vi "G#Object_GenericCreate.vi"(0 "class path":path, 2 "control names":string[](array[string]), 3 "control values":variant[](array[variant]), 4 "timeout in ms (-1)":i32=-1, 5 "error in (no error)":errorcluster, 6 "keep constructor VI ref open? (T)":bool=TRUE, 7 "respond to create event? (T)":bool=TRUE) -> (12 "constructor VI ref":refnum<vi>, 14 "reference out":refnum<class "G#Object.lvclass">, 19 "error out":errorcluster)   [LabVIEW 2020, in "G#Object.lvclass"]
doc: "Creates an instance of the class specified by the path. The path could either be directly to the constructor method, the .lvclass file or to the class folder. It is also possible to set the constructor input parameters by the \"Control Names\" and \"Control Values\" inputs.\n\nSince this function runs the constructor with VI server, making the constructor \"running top-level\", it is necessary to use the external create event in order to let this VI create the needed object and become the owner of the queues and data value reference. However, if the constructor also contains user defined queues, notifiers etc., these will be garbage collected by LabVIEW when the constructor is finished executing. To avoid this, use the Default Constructor instead.\n\nBe careful when using this VI when building executables, since paths must be correct and make sure that all needed VIs are included in the build.\n\nNote: Will not work on RT systems."
uses:
  G#Object.lvclass
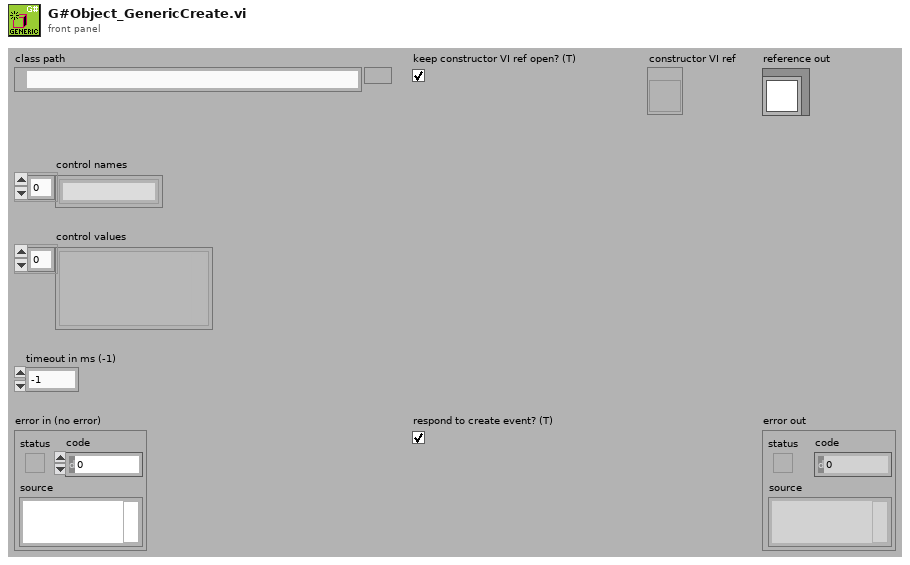
[diagram p1: front panel]
types:
  T1 = typedef "G#Object.lvclass/G#Object_EventType.ctl" = enum16{"Created new", "Looked up existing", "Deleted", "Forced delete", "Not deleted", "Garbage collected", "Cleared", "User", "Error", "External create object", "External create class attributes", "Created class attributes", "Run constructor", "Run constructor done", "Run open method", "Run open method done"}
  T2 = typedef "G#Object.lvclass/G#Object_ObjectInfoType.ctl" = cluster{"ObjectName":string, "ObjectID":u32, "Users":i32, "Counter":bool, "AttributeRefs":u32[], "FullClassName":string, "ClassName":string, "CreateMethod":T3, "GenericDestructorExists":bool, "Owner":string}
  T3 = typedef "G#Object.lvclass/G#Object_CreateMethod.ctl" = enum16{"Create", "Create or look up existing", "Look up existing"}
  T4 = enum32{"Bad", "Idle", "Run top level", "Running"}
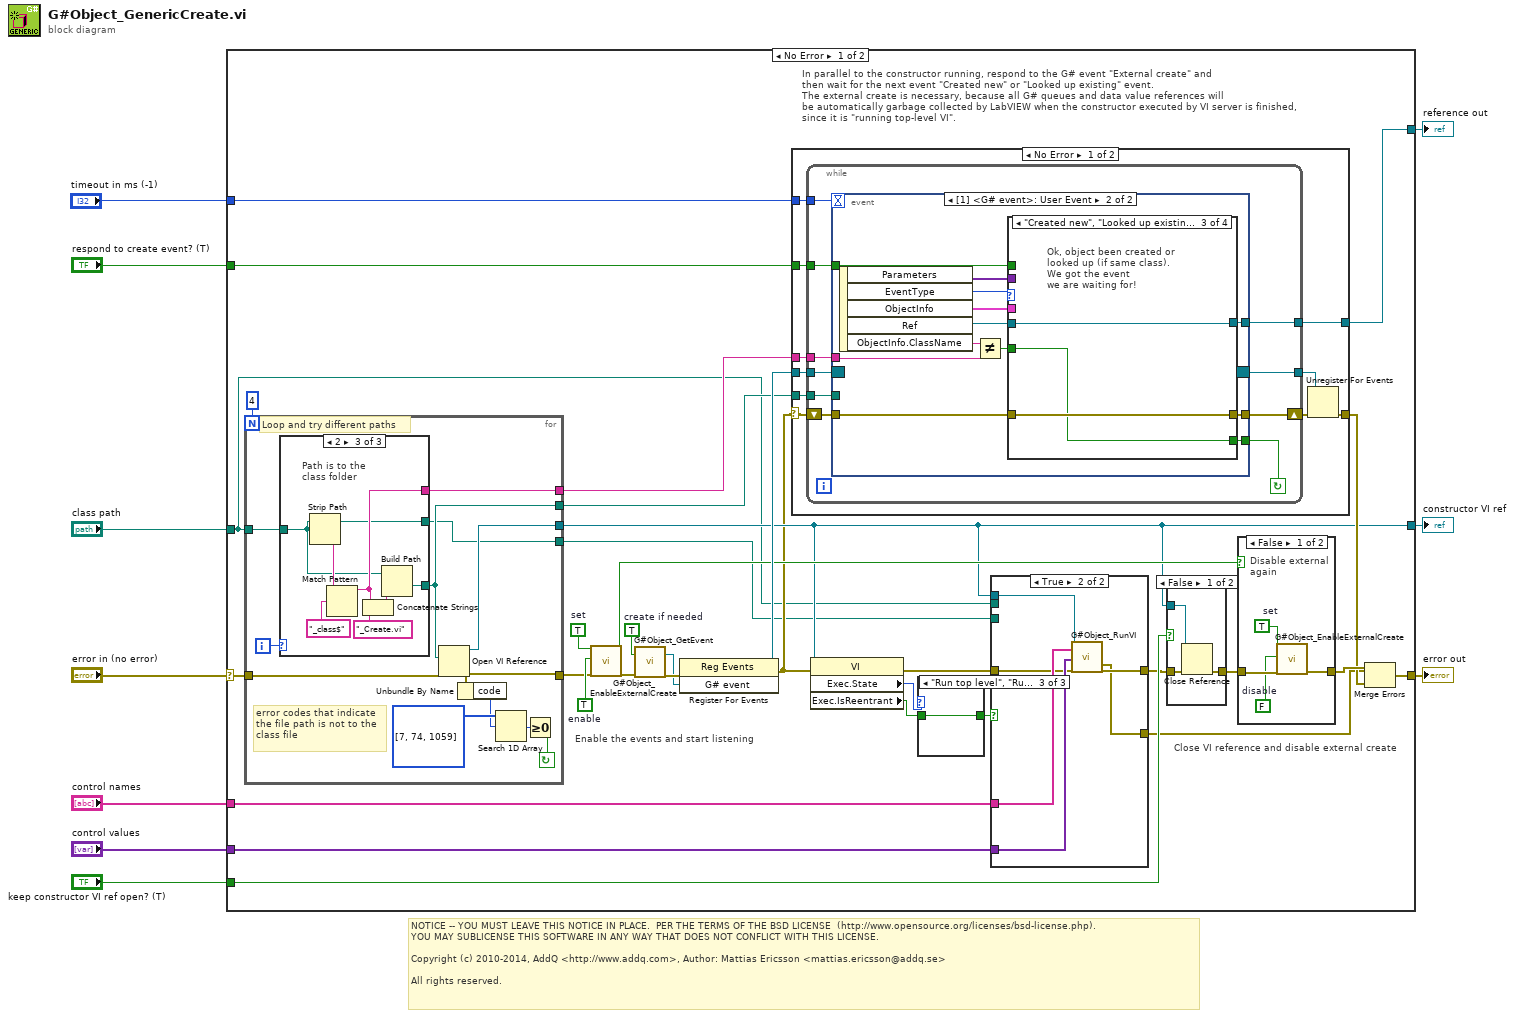
[diagram p0: block diagram]
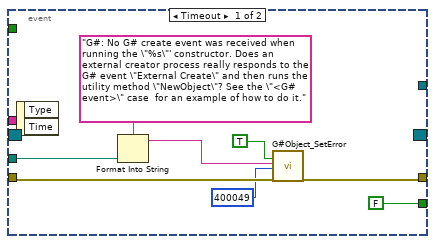
[diagram p2: hidden frame]
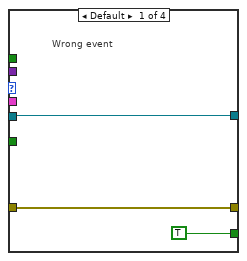
[diagram p3: hidden frame]
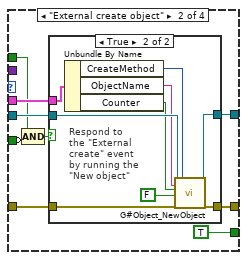
[diagram p4: hidden frame]
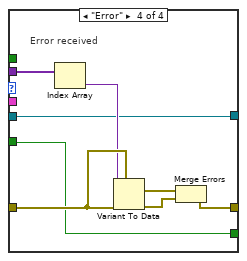
[diagram p6: hidden frame]
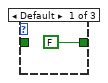
[diagram p8: hidden frame]
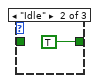
[diagram p9: hidden frame]
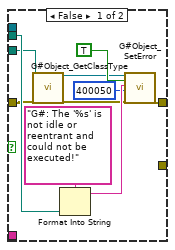
[diagram p10: hidden frame]
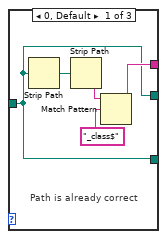
[diagram p13: hidden frame]
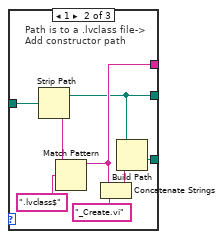
[diagram p14: hidden frame]
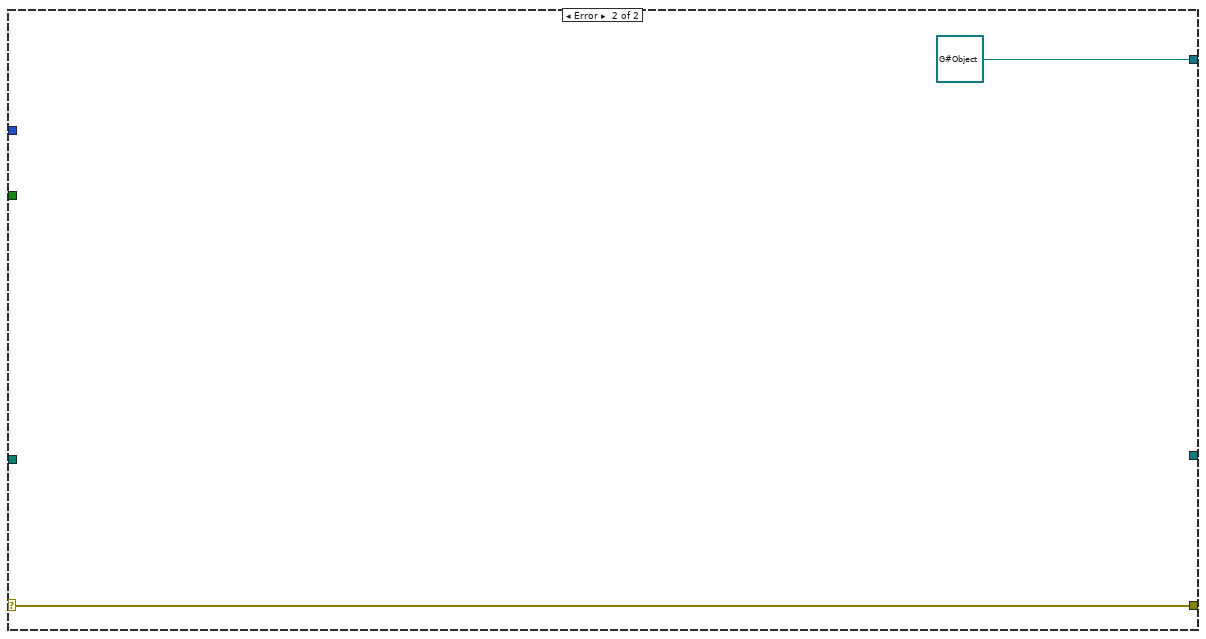
[diagram p15: hidden frame]
diagram:
  # "NOTICE -- YOU MUST LEAVE THIS NOTICE IN PLACE.  PER THE TERMS OF THE BSD LICENSE  (http://www.opensource.org/licenses/bsd-license.php).\nYOU MAY SUBLICENSE THIS SOFTWARE IN ANY WAY THAT DOES NOT CONFLICT WITH THIS LICENSE.\n\nCopyright (c) 2010-2014, AddQ <http://www.addq.com>, Author: Mattias Ericsson <mattias.ericsson@addq.se>\n\nAll rights reserved."
  n1 = case shown="No Error" "error in (no error)" {
    selector: "error in (no error)" -> [w25 w180]
    tunnel: [w36 w180] -> w9
    tunnel: [w37 refnum<class "G#Object.lvclass"> refnum ("reference in (for type)")] -> w8
    tunnel: "control names" -> [w43 _]
    tunnel: "control values" -> [w42 _]
    tunnel: "class path" -> [w12 _]
    tunnel: "keep constructor VI ref open? (T)" -> [w35 _]
    tunnel: [w19 _] -> w3
    tunnel: "respond to create event? (T)" -> [w34 _]
    tunnel: "timeout in ms (-1)" -> [w14 _]
    frame No Error {
      w31 = TRUE  # enable
      w32 = TRUE  # set
      w28 = TRUE  # create if needed
      # "Enable the events and start listening"
      # "Close VI reference and disable external create"
      # "In parallel to the constructor running, respond to the G# event \"External create\" and\nthen wait for the next event \"Created new\" or \"Looked up existing\" event.\nThe external create is necessary, because all G# queues and data value references will\nbe automatically garbage collected by LabVIEW when the constructor executed by VI server is finished,\nsince it is \"running top-level VI\"."
      n2 = for {
        N: 4 -> [_]
        tunnel: w12 -> [w157]
        tunnel: [w156] -> w19
        tunnel: [w155] -> w15
        tunnel: [w154] -> w27
        tunnel: [w147] -> w26
        tunnel: w25 -> [w153]
        tunnel: [w152] -> w11
        i -> [w158]
        stop <- w148 continue-if-true
        # "error codes that indicate\nthe file path is not to the\nclass file"
        # "Loop and try different paths"
        n3 = case shown="2" w158 {
          tunnel: w157 -> [w159 w171 w172]
          tunnel: [w159 w166 w174] -> w155
          tunnel: [w160 w165 w173] -> w154
          tunnel: [w159 w164 w172] -> w152
          frame 0, Default {
            # "Path is already correct"
            n4 = Strip Path(path=w159) -> (stripped path=w161:path)  [unwired: 1 out]
            n5 = Strip Path(path=w161) -> (name=w163:string)  [unwired: 1 out]
            n6 = Match Pattern(string=w163, regular expression="_class$") -> (before substring=w160:string)  [unwired: 1 in, 3 out]
          }
          frame 1 {
            # "Path is to a .lvclass file->\nAdd constructor path"
            n7 = Strip Path(path=w171) -> (stripped path=w164:path, name=w170:string)
            n8 = Match Pattern(string=w170, regular expression=".lvclass$") -> (before substring=w165:string)  [unwired: 1 in, 3 out]
            n9 = Concatenate Strings(w165, "_Create.vi" ("string")) -> (w167:string)
            n10 = Build Path(base path=w164, name or relative path=w167) -> (appended path=w166:path)
          }
          frame 2 {
            # "Path is to the \nclass folder"
            n11 = Strip Path(path=w172) -> (name=w178:string)  [unwired: 1 out]
            n12 = Match Pattern(string=w178, regular expression="_class$") -> (before substring=w173:string)  [unwired: 1 in, 3 out]
            n13 = Concatenate Strings(w173, "_Create.vi" ("string")) -> (w175:string)
            n14 = Build Path(base path=w172, name or relative path=w175) -> (appended path=w174:path)
          }
        }
        n15 = Open VI Reference(vi path=w155, error in (no error)=w153) -> (vi reference=w156:refnum<vi>, error out=w147:errorcluster)  [unwired: 4 in]
        n16 = Unbundle By Name(w147) -> ("code"=w149:i32)
        n17 = Search 1D Array(1D array=i32[] [7, 74, 1059], element=w149) -> (index of element=w151:i32)  [unwired: 1 in]
        n18 = Greater Or Equal To 0?(x=w151) -> (x >= 0?=w148:bool)
      }
      n19 = call "G#Object_EnableExternalCreate.vi"("set (F)"=w32, "external create enable (F)"=w31, "error in (no error)"=w26) -> ("already enabled"=w29:bool, "error out"=w33:errorcluster)  [unwired: 14 in, 1 out]
      n20 = call "G#Object_GetEvent.vi"("create if needed (T)"=w28, "error in (no error)"=w33) -> ("G# event"=w39:refnum<user-event>, "error out"=w40:errorcluster)  [unwired: 13 in, 3 out]
      n21 = register-events(error in=w40, w39) -> (reference out=w38:refnum<event-registration>, error out=w13:errorcluster)  [unwired: 1 in]
      n22 = case shown="No Error" w13 {
        selector: w13 -> [w44 w118]
        tunnel: w38 -> [w53 _]
        tunnel: [w52 _] -> w37
        tunnel: w34 -> [w49 _]
        tunnel: w27 -> [w48 _]
        tunnel: [w47 w118] -> w23
        tunnel: w15 -> [w46 _]
        tunnel: w14 -> [w45 _]
        frame No Error {
          n23 = while {
            tunnel: w53 -> [w63]
            shift-right: [w61] -> w51
            shift-left: w44 -> [w62]
            tunnel: [w59] -> w52
            tunnel: [w58] -> w50
            tunnel: w49 -> [w57]
            tunnel: w46 -> [w56]
            tunnel: w48 -> [w55]
            tunnel: w45 -> [w54]
            stop <- w60 continue-if-true
            n24 = event shown="[1] <G# event>: User Event" {
              selector: w63 -> [_ _]
              dyn-events: [_ _] -> w58
              timeout: w54 -> [_ _]
              tunnel: w62 -> [w69 w82]
              tunnel: [w70 w79] -> w61
              tunnel: [FALSE w78] -> w60
              tunnel: [_ w77] -> w59
              tunnel: w57 -> [_ w76]
              tunnel: w56 -> [w65 _]
              tunnel: w55 -> [_ w74]
              event Timeout {
                n25 = event-data() -> ()  [unwired: 1 in, 2 out]
                n26 = Format Into String(format string="G#: No G# create event was received when running the \"%s\"' constructor. Does an external creator process really responds to the G# event \"External Create\" and then runs the utility method \"NewObject\"? See the \"<G# event>\" case  for an example of how to do it." ("source"), w65) -> (resulting string=w66:string)  [unwired: 2 in, 1 out]
                n27 = call "G#Object_SetError.vi"("error (F)"=TRUE ("error"), "source"=w66, "code"=400049, "error in (no error)"=w69) -> ("error out"=w70:errorcluster)  [unwired: 15 in]
              }
              event User Event {
                n28 = event-data() -> ("Parameters"=w72:variant[], "EventType"=w83:T1, "ObjectInfo"=w81:T2, "Ref"=w80:refnum<class "G#Object.lvclass">, "ObjectInfo.ClassName"=w75:string)  [unwired: 1 in]
                n29 = Not Equal?(x=w75, y=w74) -> (x != y?=w73:bool)
                n30 = case shown="\"Created new\", \"Looked up existing\"" w83 {
                  tunnel: w82 -> [w85 w95 w109 w117]
                  tunnel: w81 -> [_ w92 _ _]
                  tunnel: w80 -> [w86 w91 w108 w111]
                  tunnel: [w85 w94 w109 w114] -> w79
                  tunnel: [TRUE TRUE w107 w110] -> w78
                  tunnel: [w86 w90 w108 w111] -> w77
                  tunnel: w76 -> [_ w88 _ _]
                  tunnel: w73 -> [_ w89 w107 w110]
                  tunnel: w72 -> [_ _ _ w116]
                  frame Default {
                    # "Wrong event"
                  }
                  frame "External create object" {
                    n31 = Compound Arithmetic op=AND(w88, invert w89) -> (w87:bool)
                    n32 = case shown="True" w87 {
                      tunnel: w95 -> [w96 w106]
                      tunnel: [w96 w105] -> w94
                      tunnel: w92 -> [_ w104]
                      tunnel: w91 -> [w97 w103]
                      tunnel: [w97 w102] -> w90
                      frame False {
                        # "Don't respond to external\ncreate event"
                      }
                      frame True {
                        # "Respond to\nthe \"External\ncreate\" event\nby running the\n\"New object\""
                        n33 = Unbundle By Name(w104) -> ("CreateMethod"=w101:T3, "ObjectName"=w100:string, "Counter"=w99:bool)
                        n34 = call "G#Object_NewObject.vi"("reference in"=w103, "object name (\"\")"=w100, "user counter (T)"=w99, "no registration (F)"=FALSE ("no registration"), "error in (no error)"=w106, "create method"=w101) -> ("reference out"=w102:refnum<class "G#Object.lvclass">, "error out"=w105:errorcluster)  [unwired: 11 in, 1 out]
                      }
                    }
                  }
                  frame "Created new", "Looked up existing" {
                    # "Ok, object been created or \nlooked up (if same class).\nWe got the event\nwe are waiting for!"
                  }
                  frame "Error" {
                    # "Error received"
                    n35 = Index Array(array=w116) -> (element=w115:variant)  [unwired: 1 in]
                    n36 = Variant To Data(error in=w117, type=w117, Variant=w115) -> (data=w112:errorcluster, error out=w113:errorcluster)
                    n37 = Merge Errors(w112, w113) -> (w114:errorcluster)
                  }
                }
              }
            }
          }
          n38 = Unregister For Events(event registration refnum=w50, error in=w51) -> (error out=w47:errorcluster)
        }
        frame Error {
        }
      }
      n39 = property class="VI"(reference=w19, error in=w13) -> (error out=w22:errorcluster, "Exec.State"=w18:T4, "Exec.IsReentrant"=w16:bool)  [unwired: 1 out]
      n40 = case shown="\"Run top level\", \"Running\"" w18 {
        tunnel: [FALSE TRUE w121] -> w17
        tunnel: w16 -> [_ _ w121]
        frame Default {
        }
        frame "Idle" {
        }
        frame "Run top level", "Running" {
        }
      }
      n41 = case shown="True" w17 {
        tunnel: w43 -> [_ w137]
        tunnel: w42 -> [_ w136]
        tunnel: w22 -> [w125 w135]
        tunnel: [w131 w134] -> w21
        tunnel: [_ w133] -> w20
        tunnel: w19 -> [_ w132]
        tunnel: w12 -> [w128 _]
        tunnel: w11 -> [w123 _]
        frame False {
          n42 = call "G#Object_GetClassType.vi"("class path"=w123, "error in (no error)"=w125) -> ("reference out"=w122:refnum<class "G#Object.lvclass">, "error out"=w124:errorcluster)  [unwired: 16 in]
          n43 = Format Into String(format string="G#: The '%s' is not idle or reentrant and could not be executed!", w128) -> (resulting string=w127:string)  [unwired: 2 in, 1 out]
          n44 = call "G#Object_SetError.vi"("reference in"=w122, "error (F)"=TRUE ("error"), "source"=w127, "code"=400050, "error in (no error)"=w124) -> ("error out"=w131:errorcluster)  [unwired: 14 in]
        }
        frame True {
          n45 = call "G#Object_RunVI.vi"("vi reference"=w132, "control names"=w137, "control values"=w136, "error in (no error)"=w135) -> ("error out from VI"=w133:errorcluster, "error out"=w134:errorcluster)  [unwired: 14 in]
        }
      }
      n46 = case shown="False" w35 {
        tunnel: w21 -> [w145 w146]
        tunnel: w19 -> [w143 _]
        tunnel: [w144 w146] -> w30
        frame False {
          n47 = Close Reference(reference=w143, error in (no error)=w145) -> (error out=w144:errorcluster)
        }
        frame True {
        }
      }
      n48 = case shown="False" w29 {
        tunnel: w30 -> [w140 w142]
        tunnel: [w141 w142] -> w24
        frame False {
          w138 = FALSE  # disable
          w139 = TRUE  # set
          # "Disable external\nagain"
          n49 = call "G#Object_EnableExternalCreate.vi"("set (F)"=w139, "external create enable (F)"=w138, "error in (no error)"=w140) -> ("error out"=w141:errorcluster)  [unwired: 14 in, 2 out]
        }
        frame True {
          # "External create\nwas enable before\ndon't disable"
        }
      }
      n50 = Merge Errors(w24, w20, w23) -> (w36:errorcluster)
    }
    frame Error {
    }
  }
  "error out" <- w9
  "reference out" <- w8
  "constructor VI ref" <- w3
